vi "Timed Messaging_Stop.vi"(9 "expected":i32=5, 10 "notification":T1=enum."Send next copy now and stop all further copies") -> (3 "Pass?":bool)   [LabVIEW 2020]
uses:
  Core/ActorFramework/Message Queue/Message Queue.lvclass
  Core/ActorFramework/Message Dequeuer/Message Dequeuer.lvclass
  Core/ActorFramework/Message/Message.lvclass
  <vilib>/ActorFramework/Time-Delayed Send Message/Time-Delay Override Options.ctl
panel:
  out "Array":refnum<class "Message.lvclass">[](array[class])
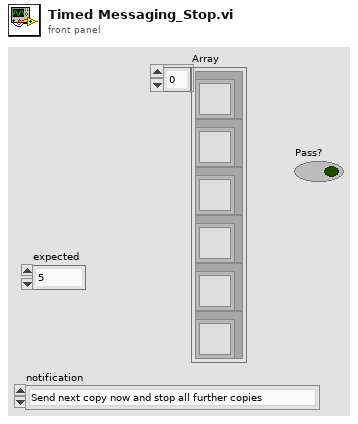
[diagram p1: front panel]
types:
  T1 = typedef "Time-Delay Override Options.ctl" = enum16{"Send next copy now", "Skip next scheduled copy", "Send next copy now and stop all further copies", "Stop all further copies"}
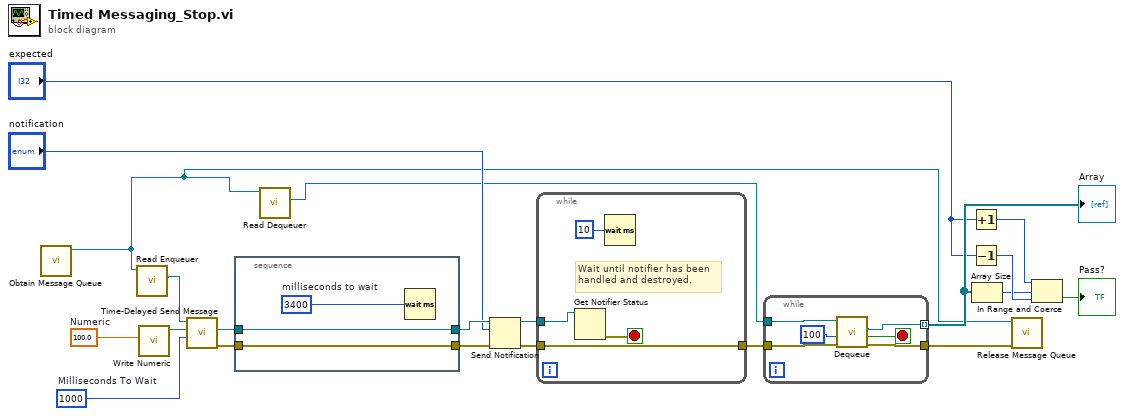
[diagram p0: block diagram]
diagram:
  w19 = 1000  # Milliseconds To Wait
  w21 = 100.0  # Numeric
  n1 = call "Obtain Message Queue.vi"() -> ("Message Queue"=w2:refnum<class "Message Queue.lvclass">)  [unwired: 10 in, 1 out]
  n2 = call "Read Enqueuer.vi"("Message Queue"=w2) -> ("Message Enqueuer"=w4:refnum<class "Message Enqueuer.lvclass">)  [unwired: 10 in]
  n3 = call "Write Numeric.vi"("Numeric"=w21) -> ("Increment Msg out"=w20:refnum<class "Increment Msg.lvclass">)  [unwired: 10 in]
  n4 = call <vilib>:"Time-Delayed Send Message.vi"("Milliseconds To Wait"=w19, "Message"=w20, "Message Enqueuer"=w4) -> ("error out"=w15:errorcluster, "Delivery Notifier"=w18:refnum<notifier>)  [unwired: 7 in]
  n5 = stacked-sequence {
    tunnel: w18 -> [w23]
    tunnel: [w23] -> w17
    tunnel: [w22] -> w16
    tunnel: w15 -> [w22]
    frame #0 {
      w24 = u32 3400  # milliseconds to wait
      n6 = Wait (ms)(milliseconds to wait=w24) -> ()  [unwired: 1 out]
    }
  }
  n7 = call "Read Dequeuer.vi"("Message Queue"=w2) -> ("Message Dequeuer"=w3:refnum<class "Message Dequeuer.lvclass">)  [unwired: 10 in]
  n8 = Send Notification(notification="notification", notifier=w17, error in (no error)=w16) -> (notifier out=w13:refnum<notifier>, error out=w12:errorcluster)
  n9 = while {
    tunnel: w13 -> [w28]
    tunnel: [w26] -> w11
    tunnel: w12 -> [w26]
    stop <- w27 stop-if-true
    # "Wait until notifier has been\nhandled and destroyed."
    n10 = Get Notifier Status(notifier=w28) -> (error out=w27:errorcluster)  [unwired: 1 in, 4 out]
    n11 = Wait (ms)(milliseconds to wait=u32 10) -> ()  [unwired: 1 out]
  }
  n12 = while {
    tunnel: w3 -> [w33]
    tunnel: w11 -> [w31]
    tunnel: [w29] -> w10 mode=indexing
    tunnel: [w30] -> w1
    stop <- w34 stop-if-true
    n13 = call "Dequeue.vi"("error in (no error)"=w31, "timeout in ms (-1)"=100, "Message Dequeuer in"=w33) -> ("error out"=w30:errorcluster, "timed out?"=w34:bool, "Message"=w29:refnum<class "Message.lvclass">)  [unwired: 4 in, 2 out]
  }
  "Array" <- w10
  n14 = Increment(x="expected") -> (x+1=w9:i32)
  n15 = Decrement(x="expected") -> (x-1=w7:i32)
  n16 = Array Size(array=w10) -> (size(s)=w6:i32)
  n17 = call "Release Message Queue.vi"("error in (no error)"=w1, "Message Queue"=w2) -> ()  [unwired: 8 in, 2 out]
  n18 = In Range and Coerce(upper limit=w9, x=w6, lower limit=w7) -> (In Range?=→"Pass?":bool)  [unwired: 1 out]
